vi "ReversedSolution.vi"(11 "Array":string[](array[string])) -> (3 "Array 2":string[](array[string]))   [LabVIEW 2019]
doc: "Generates a tab of command which is composed of the opposite moves of the tab given in entry. This allows to unshuffle a tab."
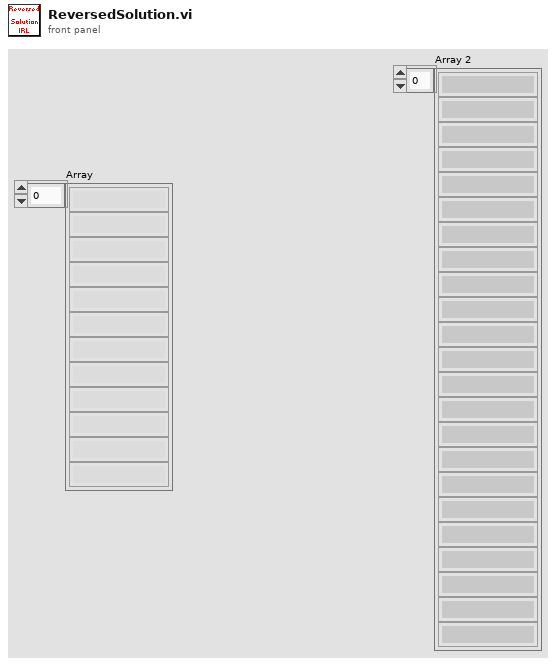
[diagram p1: front panel]
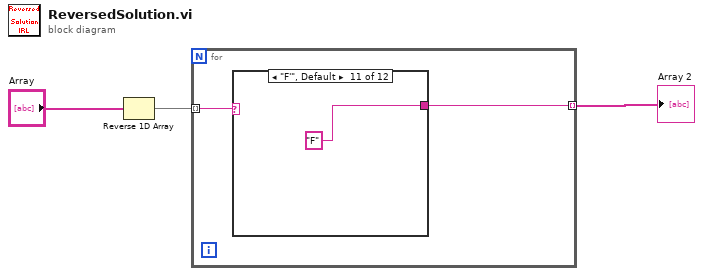
[diagram p0: block diagram]
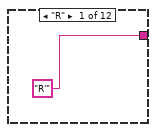
[diagram p2: hidden frame]
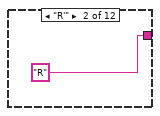
[diagram p3: hidden frame]
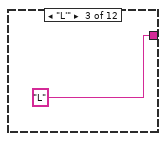
[diagram p4: hidden frame]
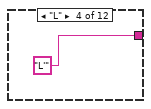
[diagram p5: hidden frame]
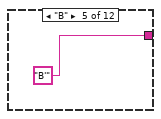
[diagram p6: hidden frame]
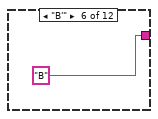
[diagram p7: hidden frame]
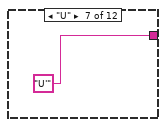
[diagram p8: hidden frame]
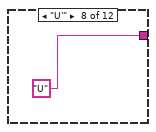
[diagram p9: hidden frame]
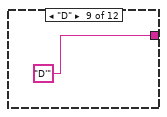
[diagram p10: hidden frame]
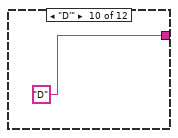
[diagram p11: hidden frame]
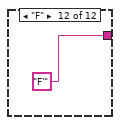
[diagram p12: hidden frame]
diagram:
  n1 = Reverse 1D Array(array="Array") -> (reversed array=w2:string[])
  n2 = for {
    tunnel: w2 -> [w5] mode=indexing
    tunnel: [w4] -> w1 mode=indexing
    n3 = case shown="\"F'\", Default" w5 {
      tunnel: ["R'" "R" "L" "L'" "B'" "B" "U'" "U" "D'" "D" "F" "F'"] -> w4
      frame "R" {
      }
      frame "R'" {
      }
      frame "L'" {
      }
      frame "L" {
      }
      frame "B" {
      }
      frame "B'" {
      }
      frame "U" {
      }
      frame "U'" {
      }
      frame "D" {
      }
      frame "D'" {
      }
      frame "F'", Default {
      }
      frame "F" {
      }
    }
  }
  "Array 2" <- w1
